vi "Hightlight Listbox.vi"(7 "Count Ref":refnum<vi>, 8 "error in (no error)":errorcluster, 9 "From DLL":string[](array[string]), 10 "From SDF":string[](array[string]), 11 "Listbox Ref":refnum<vi>) -> (0 "error out":errorcluster)   [LabVIEW 2016, in "System Mapping Tool.lvlib"]
uses:
  System Mapping Tool.lvlib
  <userlib>/_OpenG.lib/array/array.llb/Sort 1D Array (String)__ogtk.vi
  <userlib>/_OpenG.lib/array/array.llb/Reorder 1D Array2 (String)__ogtk.vi
  <userlib>/_OpenG.lib/array/array.llb/Remove Duplicates from 1D Array (String)__ogtk.vi
  <userlib>/_OpenG.lib/array/array.llb/Filter 1D Array (String)__ogtk.vi
  <userlib>/_OpenG.lib/array/array.llb/Reorder 1D Array2 (I32)__ogtk.vi
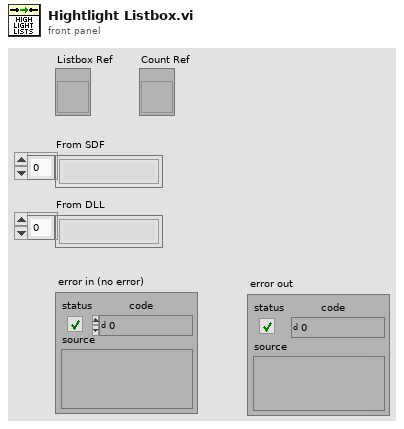
[diagram p1: front panel]
types:
  T1 = enum8{"Enabled", "Disabled", "Disabled and Grayed Out"}
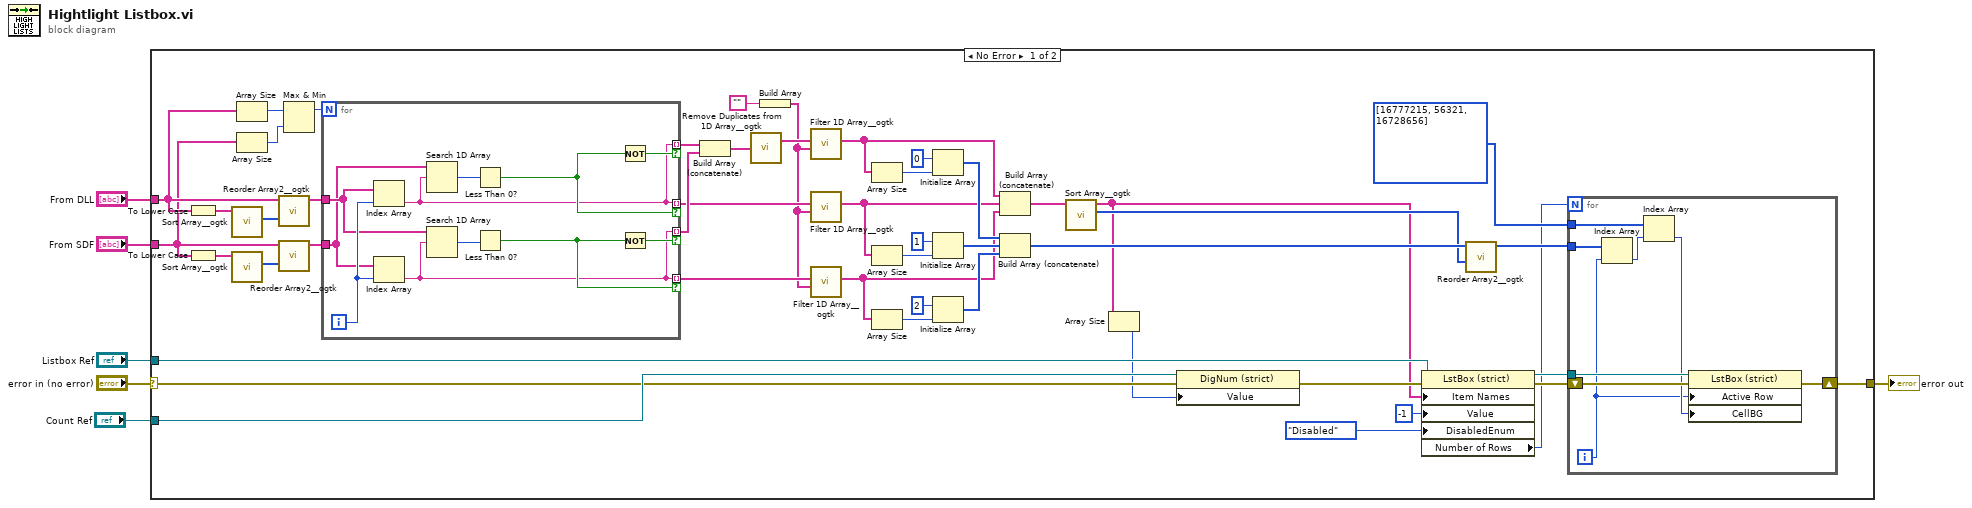
[diagram p0: block diagram]
diagram:
  n1 = case shown="No Error" "error in (no error)" {
    selector: "error in (no error)" -> [w10 w74]
    tunnel: "From DLL" -> [w46 _]
    tunnel: "From SDF" -> [w42 _]
    tunnel: [w24 w74] -> w3
    tunnel: "Listbox Ref" -> [w21 _]
    tunnel: "Count Ref" -> [w11 _]
    frame No Error {
      n2 = To Lower Case(string=w46) -> (all lower case string=w44:string[])
      n3 = To Lower Case(string=w42) -> (all lower case string=w41:string[])
      n4 = call-poly <userlib>:"Sort Array__ogtk.vi"("Array in"=w44) -> ("Sorted Pointers"=w45:i32[])  [unwired: 9 in, 1 out]
      n5 = call-poly <userlib>:"Sort Array__ogtk.vi"("Array in"=w41) -> ("Sorted Pointers"=w43:i32[])  [unwired: 9 in, 1 out]
      n6 = Array Size(array=w46) -> (size(s)=w53:i32)
      n7 = Array Size(array=w42) -> (size(s)=w52:i32)
      n8 = call-poly <userlib>:"Reorder Array2__ogtk.vi"("indices"=w45, "array"=w46) -> ("reordered array"=w48:string[])  [unwired: 9 in]
      n9 = call-poly <userlib>:"Reorder Array2__ogtk.vi"("indices"=w43, "array"=w42) -> ("reordered array"=w47:string[])  [unwired: 9 in]
      n10 = Max & Min(x=w53, y=w52) -> (max(x,y)=w54:i32)  [unwired: 1 out]
      n11 = for {
        N: w54 -> [_]
        tunnel: w48 -> [w72]
        tunnel: w47 -> [w71]
        tunnel: [w64] -> w16 mode=indexing if=w67
        tunnel: [w63] -> w14 mode=indexing if=w68
        tunnel: [w63] -> w50 mode=indexing if=w66
        tunnel: [w64] -> w51 mode=indexing if=w65
        i -> [w73]
        n12 = Index Array(array=w72, index=w73) -> (element=w64:string)
        n13 = Index Array(array=w71, index=w73) -> (element=w63:string)
        n14 = Search 1D Array(1D array=w71, element=w64) -> (index of element=w70:i32)  [unwired: 1 in]
        n15 = Search 1D Array(1D array=w72, element=w63) -> (index of element=w69:i32)  [unwired: 1 in]
        n16 = Less Than 0?(x=w70) -> (x < 0?=w67:bool)
        n17 = Less Than 0?(x=w69) -> (x < 0?=w68:bool)
        n18 = Not(x=w67) -> (.not. x?=w65:bool)
        n19 = Not(x=w68) -> (.not. x?=w66:bool)
      }
      n20 = Build Array (concatenate)(w51, w50) -> (w49:string[])
      n21 = call-poly <userlib>:"Remove Duplicates from 1D Array__ogtk.vi"("Input Array"=w49) -> ("Output Array"=w19:string[])  [unwired: 1 out]
      n22 = Build Array("") -> (w12:string[])
      n23 = call-poly <userlib>:"Filter 1D Array__ogtk.vi"("items to filter"=w12, "array"=w19) -> ("filtered array"=w17:string[])  [unwired: 4 in, 1 out]
      n24 = call-poly <userlib>:"Filter 1D Array__ogtk.vi"("items to filter"=w12, "array"=w16) -> ("filtered array"=w15:string[])  [unwired: 4 in, 1 out]
      n25 = call-poly <userlib>:"Filter 1D Array__ogtk.vi"("items to filter"=w12, "array"=w14) -> ("filtered array"=w13:string[])  [unwired: 4 in, 1 out]
      n26 = Array Size(array=w17) -> (size(s)=w40:i32)
      n27 = Array Size(array=w15) -> (size(s)=w37:i32)
      n28 = Array Size(array=w13) -> (size(s)=w36:i32)
      n29 = Initialize Array(0, w40) -> (w33:i32[])
      n30 = Initialize Array(1, w37) -> (w34:i32[])
      n31 = Initialize Array(2, w36) -> (w32:i32[])
      n32 = Build Array (concatenate)(w17, w15, w13) -> (w31:string[])
      n33 = Build Array (concatenate)(w33, w34, w32) -> (w30:i32[])
      n34 = call-poly <userlib>:"Sort Array__ogtk.vi"("Array in"=w31) -> ("Sorted Pointers"=w29:i32[], "Sorted Array out"=w8:string[])  [unwired: 9 in]
      n35 = Array Size(array=w8) -> (size(s)=w7:i32)
      n36 = property class="DigNum (strict)"(reference=w11, error in=w10, "Value"=w7) -> (error out=w9:errorcluster)  [unwired: 1 out]
      n37 = property class="LstBox (strict)"(reference=w21, error in=w9, "Item Names"=w8, "Value"=-1, "DisabledEnum"=T1."Disabled" ("Disabled")) -> (reference out=w26:refnum<vi>, error out=w27:errorcluster, "Number of Rows"=w20:u32)
      n38 = call-poly <userlib>:"Reorder Array2__ogtk.vi"("indices"=w29, "array"=w30) -> ("reordered array"=w28:i32[])  [unwired: 9 in]
      n39 = for {
        N: w20 -> [_]
        tunnel: w28 -> [w60]
        tunnel: w26 -> [w62]
        tunnel: u32[] [16777215, 56321, 16728656] -> [w59]
        shift-right: [w57] -> w24
        shift-left: w27 -> [w61]
        i -> [w55]
        n40 = Index Array(array=w60, index=w55) -> (element=w56:i32)
        n41 = Index Array(array=w59, index=w56) -> (element=w58:u32)
        n42 = property class="LstBox (strict)"(reference=w62, error in=w61, "Active Row"=w55, "CellBG"=w58) -> (error out=w57:errorcluster)  [unwired: 1 out]
      }
    }
    frame Error {
    }
  }
  "error out" <- w3
